vi "Program Device.vi"(5 "Tool Path":path, 7 "Firmware Path":path, 8 "error in":errorcluster, 9 "Flash Timeout (ms)":i32=50000, 10 "Com Port":string, 11 "Slide in":refnum<vi>) -> (0 "error out":errorcluster, 3 "Success":bool)   [LabVIEW 2020]
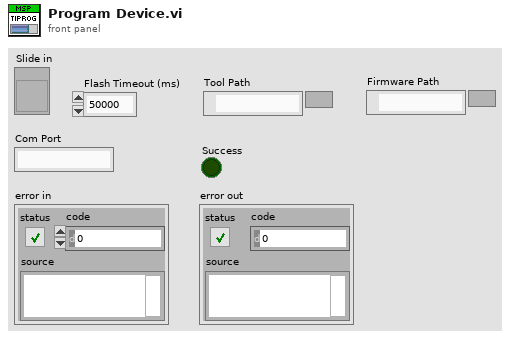
[diagram p1: front panel]
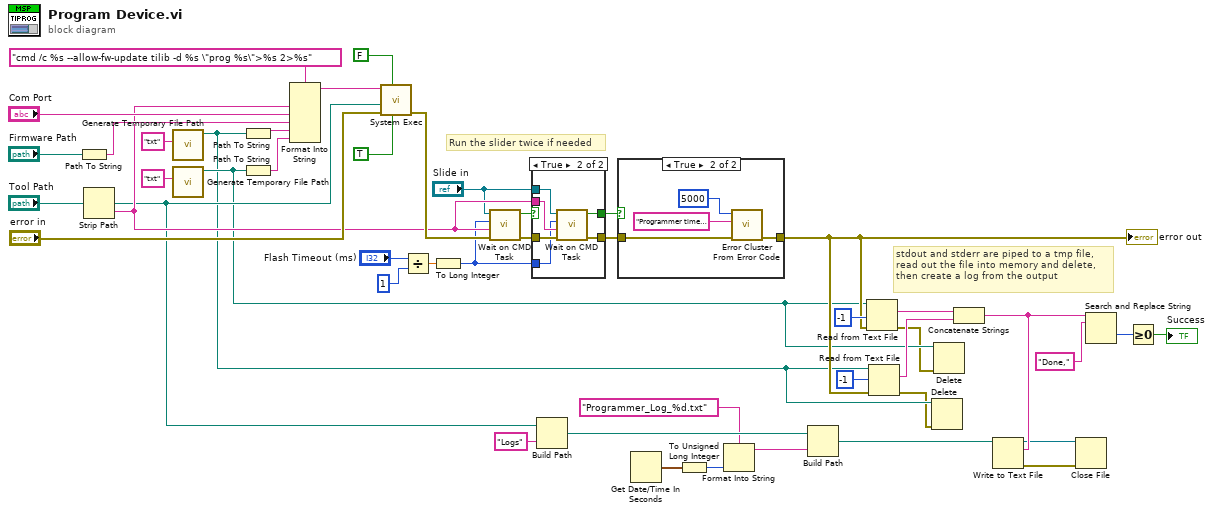
[diagram p0: block diagram]
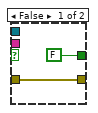
[diagram p2: hidden frame]
diagram:
  # "stdout and stderr are piped to a tmp file,\nread out the file into memory and delete,\nthen create a log from the output"
  # "Run the slider twice if needed"
  n1 = Path To String(path="Firmware Path") -> (string=w43:string)
  n2 = Strip Path(path="Tool Path") -> (stripped path=w16:path, name=w30:string)
  n3 = call <vilib>:"Generate Temporary File Path.vi"("Temporary File Extension (tmp)"="txt") -> ("Unique Temporary File Path"=w7:path)  [unwired: 9 in, 1 out]
  n4 = call <vilib>:"Generate Temporary File Path.vi"("Temporary File Extension (tmp)"="txt") -> ("Unique Temporary File Path"=w8:path)  [unwired: 9 in, 1 out]
  n5 = Path To String(path=w7) -> (string=w39:string)
  n6 = Path To String(path=w8) -> (string=w37:string)
  n7 = Format Into String(format string="cmd /c %s --allow-fw-update tilib -d %s \"prog %s\">%s 2>%s", w30, "Com Port", w43, w39, w37) -> (resulting string=w47:string)  [unwired: 2 in, 1 out]
  n8 = call <vilib>:"System Exec.vi"("run minimized? (F)"=TRUE, "wait until completion? (T)"=FALSE, "error in (no error)"="error in", "working directory"=w16, "command line"=w47) -> ("error out"=w41:errorcluster)  [unwired: 3 in, 3 out]
  n9 = Divide(x="Flash Timeout (ms)", y=1) -> (x/y=w26:dbl)
  n10 = To Long Integer(number=w26) -> (32bit integer=w25:i32)
  n11 = call "Wait on CMD Task.vi"("error in (no error)"=w41, "Programmer Name"=w30, "Flash Timeout (ms)"=w25, "Slide in"="Slide in") -> ("error out"=w34:errorcluster, "Timed out?"=w31:bool)  [unwired: 6 in]
  n12 = case shown="True" w31 {
    tunnel: w34 -> [w48 w55]
    tunnel: [w48 w54] -> w33
    tunnel: [FALSE ("Timed out?") w53] -> w32
    tunnel: w30 -> [_ w52]
    tunnel: "Slide in" -> [_ w51]
    tunnel: w25 -> [_ w50]
    frame False {
    }
    frame True {
      n13 = call "Wait on CMD Task.vi"("error in (no error)"=w55, "Programmer Name"=w52, "Flash Timeout (ms)"=w50, "Slide in"=w51) -> ("error out"=w54:errorcluster, "Timed out?"=w53:bool)  [unwired: 6 in]
    }
  }
  n14 = Build Path(base path=w16, name or relative path="Logs") -> (appended path=w14:path)
  n15 = case shown="True" w32 {
    tunnel: w33 -> [w56 w60]
    tunnel: [w56 w59] -> w18
    frame False {
    }
    frame True {
      n16 = call <vilib>:"Error Cluster From Error Code.vi"("error in (no error)"=w60, "error message (\"\")"="Programmer timed out...." ("error message (\"\")"), "error code (0)"=5000) -> ("error out"=w59:errorcluster)  [unwired: 6 in]
    }
  }
  "error out" <- w18
  n17 = Get Date/Time In Seconds() -> (seconds since 1Jan1904=w2:timestamp)
  n18 = To Unsigned Long Integer(number=w2) -> (unsigned 32bit integer=w3:u32)
  n19 = Format Into String(format string="Programmer_Log_%d.txt", w3) -> (resulting string=w13:string)  [unwired: 2 in, 1 out]
  n20 = Build Path(base path=w14, name or relative path=w13) -> (appended path=w12:path)
  n21 = Read from Text File(file (use dialog)=w8, count=-1, error in=w18) -> (text=w22:string, error out=w5:errorcluster)  [unwired: 1 in, 2 out]
  n22 = Read from Text File(file (use dialog)=w7, count=-1, error in=w18) -> (text=w21:string, error out=w6:errorcluster)  [unwired: 1 in, 2 out]
  n23 = Delete(path (use dialog)=w7, error in=w6) -> ()  [unwired: 3 in, 3 out]
  n24 = Delete(path (use dialog)=w8, error in=w5) -> ()  [unwired: 3 in, 3 out]
  n25 = Concatenate Strings(w22, w21) -> (w11:string)
  n26 = Write to Text File(file (use dialog)=w12, text=w11) -> (refnum out=w9:refnum<file>, error out=w10:errorcluster)  [unwired: 2 in, 1 out]
  n27 = Close File(refnum=w9, error in=w10) -> ()  [unwired: 2 out]
  n28 = Search and Replace String(input string=w11, search string="Done,") -> (offset past replacement=w19:i32)  [unwired: 6 in, 3 out]
  n29 = Greater Or Equal To 0?(x=w19) -> (x >= 0?=→"Success":bool)
